vi "Write Strings And Values [].vi"(5 "Strings And Values []":T1, 9 "Combobox in":refnum<class "Combobox.lvclass">) -> (3 "Combobox out":refnum<class "Combobox.lvclass">)   [LabVIEW 2014, in "Combobox.lvclass"]
uses:
  Combobox.lvclass
  <vilib>/Utility/miscctls.llb/LVComboBoxStrsAndValuesArrayTypeDef.ctl
  Combobox.lvclass/Combobox.ctl
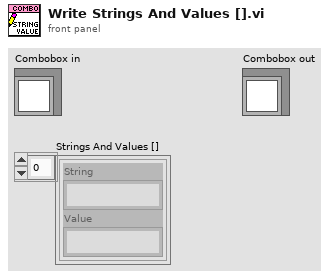
[diagram p1: front panel]
types:
  T1 = typedef "LVComboBoxStrsAndValuesArrayTypeDef.ctl" = cluster{"String":string, "Value":string}[]
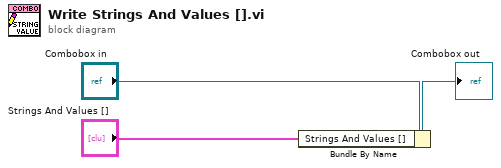
[diagram p0: block diagram]
diagram:
  n1 = Bundle By Name(cluster="Combobox in", "Strings And Values []"="Strings And Values []") -> (→"Combobox out":refnum<class "Combobox.lvclass">)
